vi "Queue Release.vi"(10 "Queue":refnum<data-value>) -> (0 "error out":errorcluster)   [LabVIEW 2021, in "jettl Queue Actor.lvlib"]
uses:
  Actor/Msg/Msg.lvclass
  jettl Queue Actor.lvlib
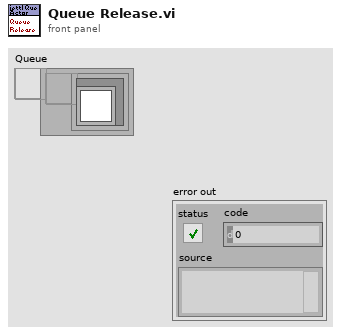
[diagram p1: front panel]
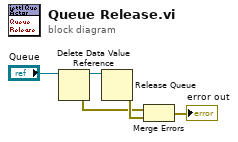
[diagram p0: block diagram]
diagram:
  n1 = Delete Data Value Reference(data value reference="Queue") -> (data value=w5:refnum<queue>, error out=w2:errorcluster)  [unwired: 1 in]
  n2 = Release Queue(queue=w5) -> (error out=w4:errorcluster)  [unwired: 2 in, 2 out]
  n3 = Merge Errors(w2, w4) -> (→"error out":errorcluster)
